vi "Biax24X setup.vi"() -> (0 "buffer size":i32=500000, 1 "Footer String":string, 2 "Channels, Hor load, Hor Disp, Vert Load, Vert Disp, LVDT1, LVDT2, LVDT3, LVDT4":string[](array[string])=["0", "1", "2", "3"], 3 "Number of Channels":i32, 4 "ASCII footer 2":bool, 5 "Device":i32=1, 6 "Channel Names":string[](array[string]), 8 "Header and Const.; Del, SR, #Scans, Write int":T1={"Delay"=-1.0, "Scan_Rate"=10000, "Number of scans"=10000, "Write time int (s)"=30} {"Delay" format="%.2f"})   [LabVIEW 2013]
doc: "This vi takes input from the operator: sets the scan rate, collects the length in inches, the sample diameter in inches, and the interchannel delay rate (default is -1.0) The vi puts out those constants along with the voltage limits for each of the data acquisition channels. The default settings are channel 0, 1 = confining and pore pressure transducer amplifiers, respectively, 0-5 volts; temperature transducer amplifier, 0-5 volts; dcdt +-3 volts (12.6 v/in); load cell after amplification: 12600 pounds force per volt."
uses:
  BiaxGlobals.vi
panel:
  in  "ASCII footer":bool=TRUE
  in  "String 23":string="Vert DCDT"
  in  "String 22":string="Vert LOAD"
  in  "String 21":string="Hor DCDT"
  in  "String 20":string="Hor LOAD"
  in  "String 19":string="Pc Disp"
  in  "String 18":string="Pc LOAD"
  in  "String 17":string="Ppa Disp"
  in  "String 16":string="Ppa LOAD"
  in  "Number of Channels":i32=4 min=1 max=8 step=1
  in  "Go on":bool
  in  "Delay":sgl=-1.0 format="%^.2e"
  out "Acquisition Rate \n(fixed at 10000 \nsamples/sec)":i32=10000
  out "Number of scans averaged for a single record output\n(while running Labview you can switch between 1, 10, 100, 1k, 10k samples/sec)":i32=10000
  in  "buffer size (500000 scans)":i32=500000
  out "write int":i32=30
  in  "Time interval to write to disk (seconds)\nNOTE: 30sec is optimal for 10 kHz sample rate":i32=30
  # "Press \"Go On\" when\nConstants are Entered\n\nDefault Delay setting \nis -1.0"
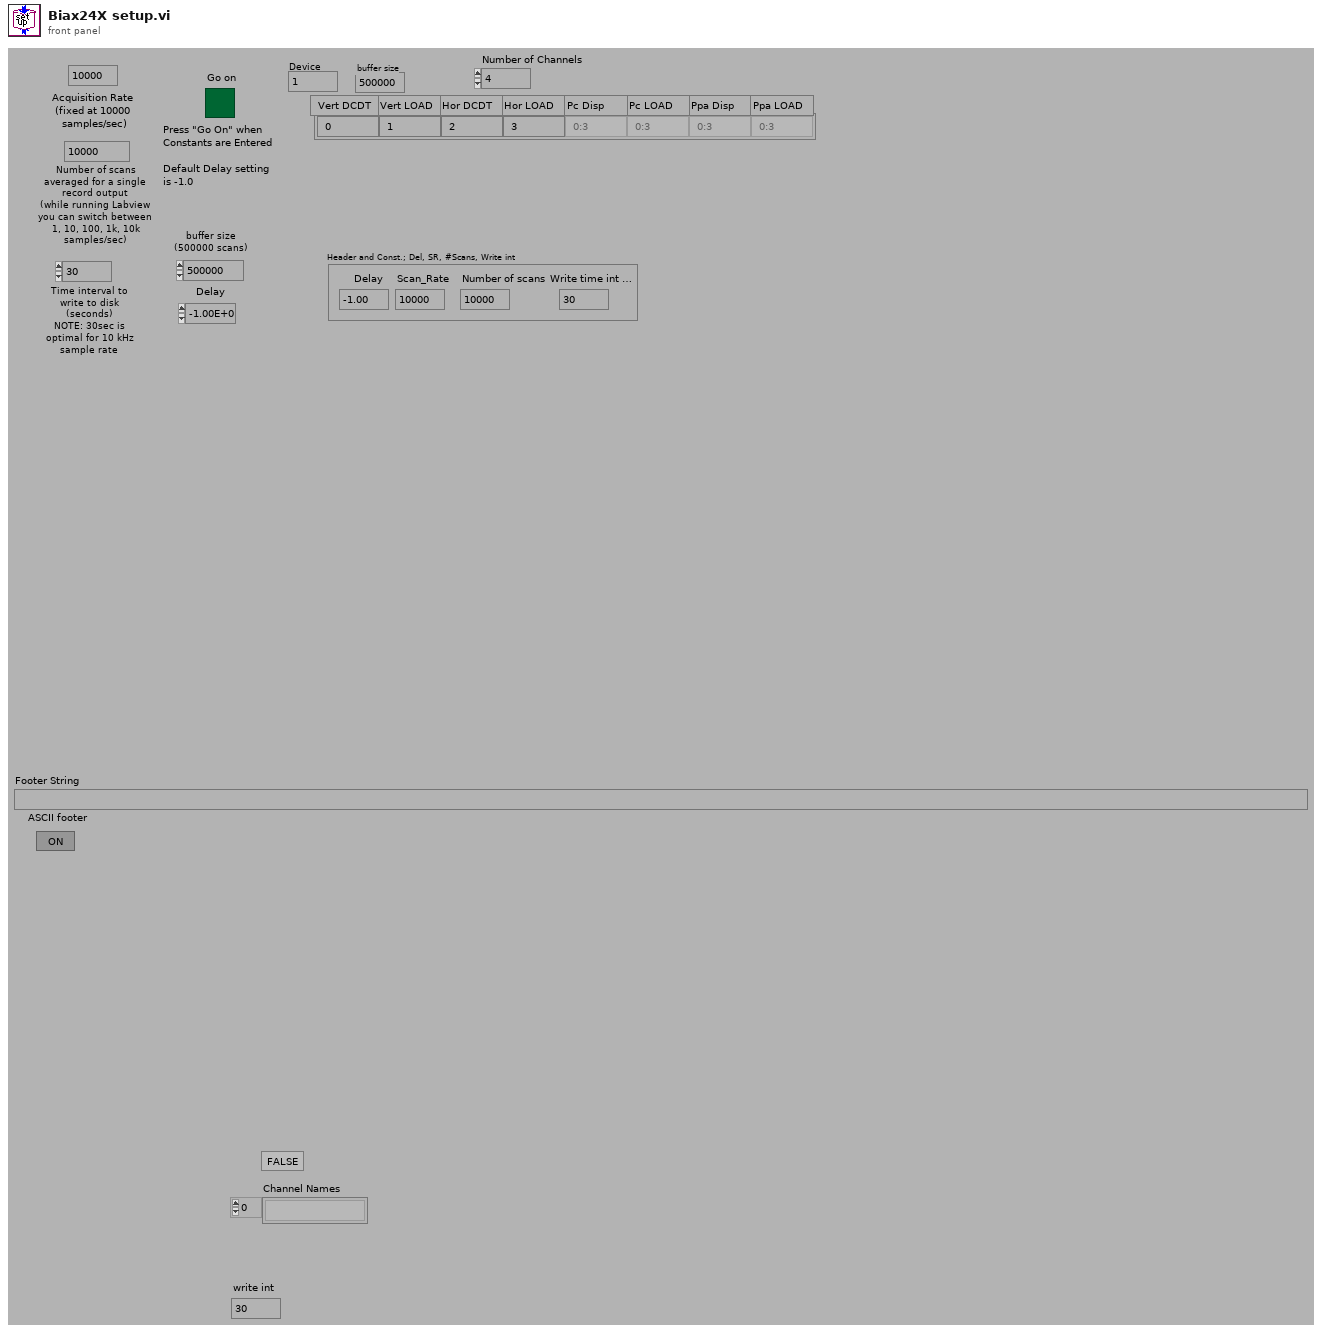
[diagram p1: front panel]
types:
  T1 = cluster{"Delay":dbl, "Scan_Rate":i32, "Number of scans":i32, "Write time int (s)":i32}
  T2 = cluster{"Delay":sgl, i32, i32, "Time interval to write to disk (seconds)\nNOTE: 30sec is optimal for 10 kHz sample rate":i32}
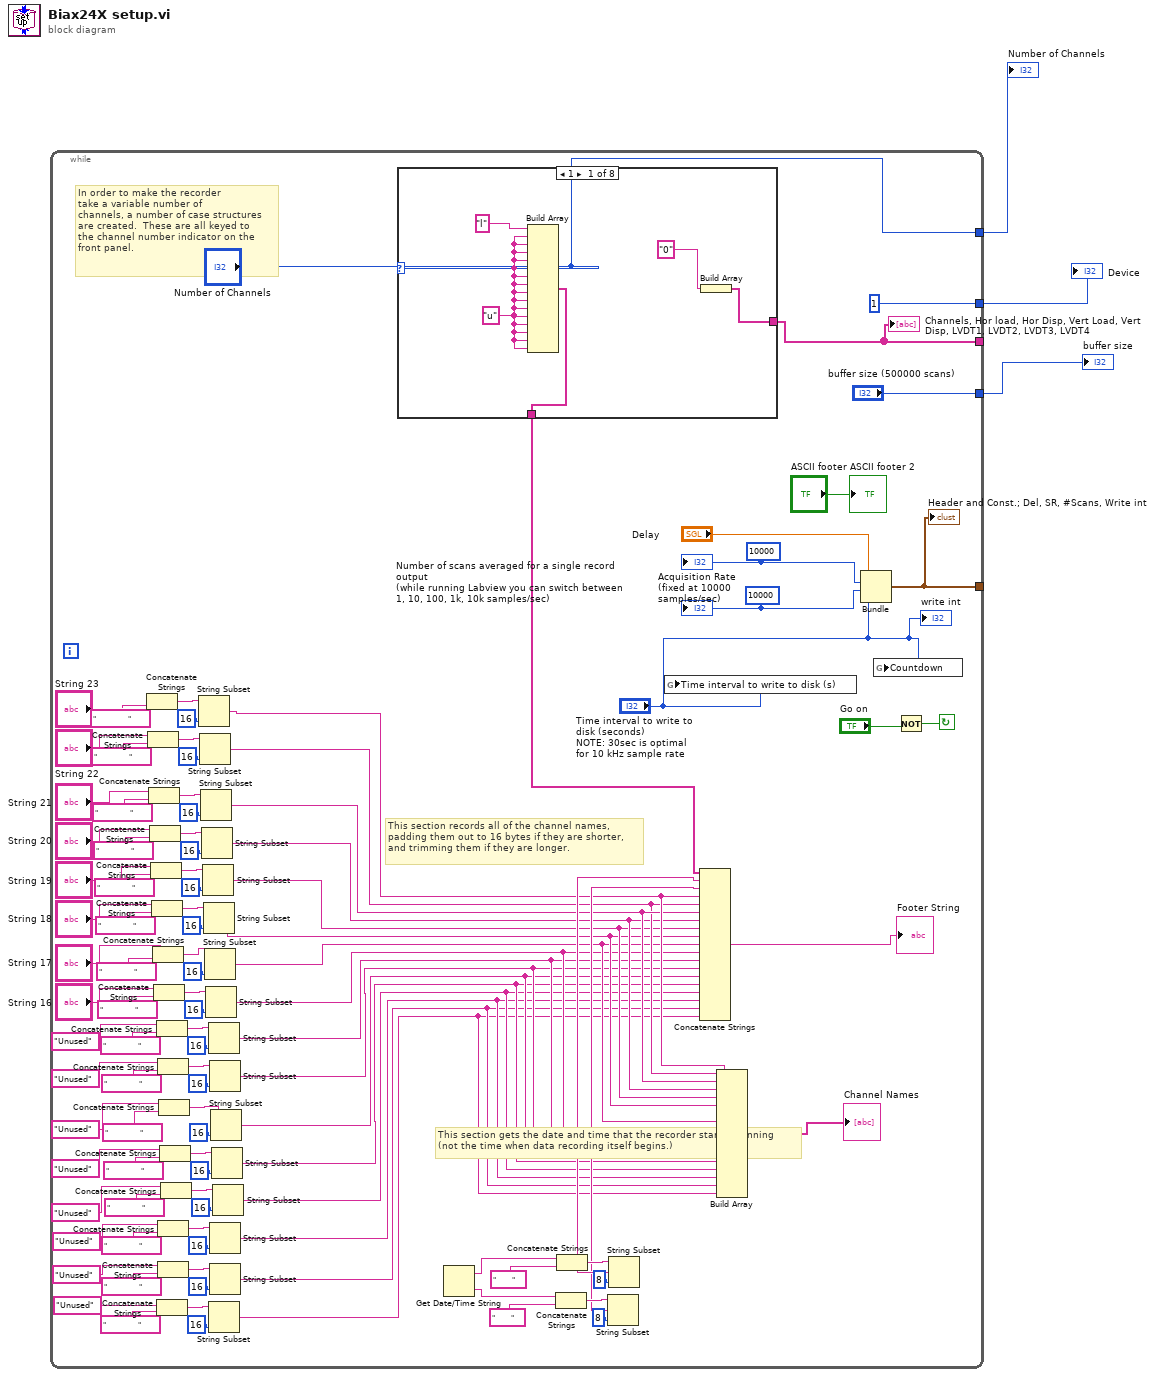
[diagram p0: block diagram]
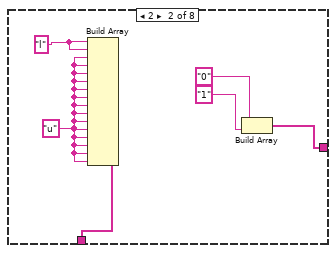
[diagram p2: hidden frame]
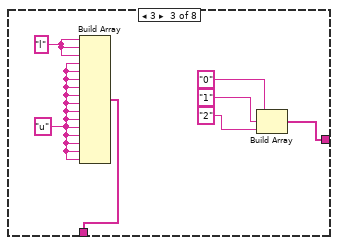
[diagram p3: hidden frame]
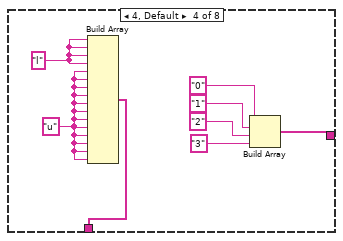
[diagram p4: hidden frame]
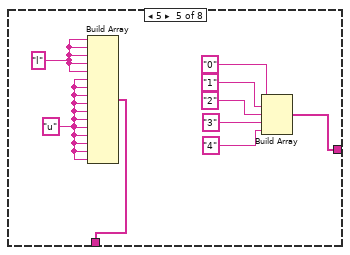
[diagram p5: hidden frame]
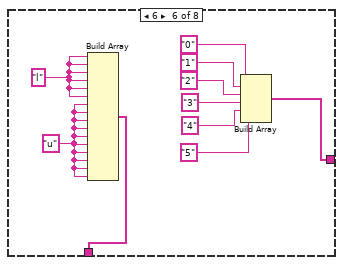
[diagram p6: hidden frame]
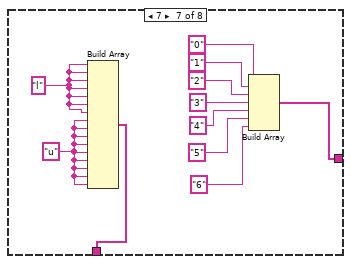
[diagram p7: hidden frame]
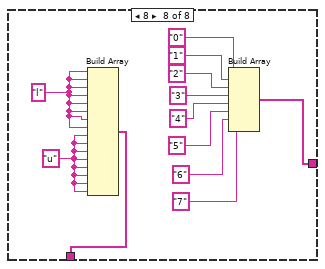
[diagram p8: hidden frame]
diagram:
  n1 = while {
    tunnel: ["buffer size (500000 scans)"] -> w3
    tunnel: [w99] -> _
    tunnel: [1] -> w2
    tunnel: [w98] -> _
    tunnel: ["Number of Channels"] -> w1
    stop <- w107 continue-if-true
    w101 = 10000
    w102 = 10000
    # "This section gets the date and time that the recorder started running \n(not the time when data recording itself begins.)"
    # "In order to make the recorder\ntake a variable number of\nchannels, a number of case structures\nare created.  These are all keyed to\nthe channel number indicator on the\nfront panel."
    # "This section records all of the channel names,\npadding them out to 16 bytes if they are shorter,\nand trimming them if they are longer."
    n2 = Concatenate Strings("String 23", "                ") -> (w95:string)
    n3 = Concatenate Strings("String 22", "                ") -> (w92:string)
    n4 = Concatenate Strings("String 21", "                ") -> (w89:string)
    n5 = Concatenate Strings("String 20", "                ") -> (w86:string)
    n6 = Concatenate Strings("String 19", "                ") -> (w83:string)
    n7 = Concatenate Strings("String 18", "                ") -> (w80:string)
    n8 = Concatenate Strings("String 17", "                ") -> (w77:string)
    n9 = Concatenate Strings("String 16", "                ") -> (w74:string)
    n10 = Concatenate Strings("Unused" ("String 24"), "                ") -> (w71:string)
    n11 = Concatenate Strings("Unused" ("String 24"), "                ") -> (w50:string)
    n12 = Concatenate Strings("Unused" ("String 24"), "                ") -> (w68:string)
    n13 = Concatenate Strings("Unused" ("String 24"), "                ") -> (w56:string)
    n14 = Concatenate Strings("Unused" ("String 24"), "                ") -> (w53:string)
    n15 = Concatenate Strings("Unused" ("String 24"), "                ") -> (w65:string)
    n16 = Concatenate Strings("Unused" ("String 24"), "                ") -> (w62:string)
    n17 = Concatenate Strings("Unused" ("String 24"), "                ") -> (w59:string)
    n18 = String Subset(string=w95, length (rest)=16 ("length (rest)")) -> (substring=w27:string)  [unwired: 1 in]
    n19 = String Subset(string=w92, length (rest)=16 ("length (rest)")) -> (substring=w25:string)  [unwired: 1 in]
    n20 = String Subset(string=w89, length (rest)=16 ("length (rest)")) -> (substring=w26:string)  [unwired: 1 in]
    n21 = String Subset(string=w86, length (rest)=16 ("length (rest)")) -> (substring=w24:string)  [unwired: 1 in]
    n22 = String Subset(string=w83, length (rest)=16 ("length (rest)")) -> (substring=w23:string)  [unwired: 1 in]
    n23 = String Subset(string=w80, length (rest)=16 ("length (rest)")) -> (substring=w22:string)  [unwired: 1 in]
    n24 = String Subset(string=w77, length (rest)=16 ("length (rest)")) -> (substring=w21:string)  [unwired: 1 in]
    n25 = String Subset(string=w74, length (rest)=16 ("length (rest)")) -> (substring=w20:string)  [unwired: 1 in]
    n26 = String Subset(string=w71, length (rest)=16 ("length (rest)")) -> (substring=w19:string)  [unwired: 1 in]
    n27 = String Subset(string=w50, length (rest)=16 ("length (rest)")) -> (substring=w12:string)  [unwired: 1 in]
    n28 = String Subset(string=w68, length (rest)=16 ("length (rest)")) -> (substring=w18:string)  [unwired: 1 in]
    n29 = String Subset(string=w56, length (rest)=16 ("length (rest)")) -> (substring=w14:string)  [unwired: 1 in]
    n30 = String Subset(string=w53, length (rest)=16 ("length (rest)")) -> (substring=w13:string)  [unwired: 1 in]
    n31 = String Subset(string=w65, length (rest)=16 ("length (rest)")) -> (substring=w17:string)  [unwired: 1 in]
    n32 = String Subset(string=w62, length (rest)=16 ("length (rest)")) -> (substring=w16:string)  [unwired: 1 in]
    n33 = String Subset(string=w59, length (rest)=16 ("length (rest)")) -> (substring=w15:string)  [unwired: 1 in]
    n34 = case shown="1" "Number of Channels" {
      tunnel: [w112 w117 w123 w134 w139 w147 w158 w168] -> w98
      tunnel: [w110 w114 w120 w127 w135 w145 w154 w167] -> w4
      frame 1 {
        w109 = "u" ("element")
        n35 = Build Array("l", w109, w109, w109, w109, w109, w109, w109, w109, w109, w109, w109, w109, w109, w109, w109) -> (w110:string[])
        n36 = Build Array("0") -> (w112:string[])
      }
      frame 2 {
        w115 = "u" ("element")
        w116 = "l"
        n37 = Build Array(w116, w116, w115, w115, w115, w115, w115, w115, w115, w115, w115, w115, w115, w115, w115, w115) -> (w114:string[])
        n38 = Build Array("0", "1") -> (w117:string[])
      }
      frame 3 {
        w121 = "u" ("element")
        w122 = "l"
        n39 = Build Array(w122, w122, w122, w121, w121, w121, w121, w121, w121, w121, w121, w121, w121, w121, w121, w121) -> (w120:string[])
        n40 = Build Array("0", "1", "2") -> (w123:string[])
      }
      frame 4, Default {
        w128 = "u" ("element")
        w129 = "l"
        n41 = Build Array(w129, w129, w129, w129, w128, w128, w128, w128, w128, w128, w128, w128, w128, w128, w128, w128) -> (w127:string[])
        n42 = Build Array("0", "1", "2", "3") -> (w134:string[])
      }
      frame 5 {
        w136 = "u" ("element")
        w137 = "l"
        n43 = Build Array(w137, w137, w137, w137, w137, w136, w136, w136, w136, w136, w136, w136, w136, w136, w136, w136) -> (w135:string[])
        n44 = Build Array("0", "1", "2", "3", "4") -> (w139:string[])
      }
      frame 6 {
        w144 = "u" ("element")
        w146 = "l"
        n45 = Build Array(w146, w146, w146, w146, w146, w146, w144, w144, w144, w144, w144, w144, w144, w144, w144, w144) -> (w145:string[])
        n46 = Build Array("0", "1", "2", "3", "4", "5") -> (w147:string[])
      }
      frame 7 {
        w155 = "u" ("element")
        w156 = "l"
        n47 = Build Array(w156, w156, w156, w156, w156, w156, w156, w155, w155, w155, w155, w155, w155, w155, w155, w155) -> (w154:string[])
        n48 = Build Array("0", "1", "2", "3", "4", "5", "6") -> (w158:string[])
      }
      frame 8 {
        w165 = "u" ("element")
        w166 = "l"
        n49 = Build Array(w166, w166, w166, w166, w166, w166, w166, w166, w165, w165, w165, w165, w165, w165, w165, w165) -> (w167:string[])
        n50 = Build Array("0", "1", "2", "3", "4", "5", "6", "7") -> (w168:string[])
      }
    }
    "Channels, Hor load, Hor Disp, Vert Load, Vert Disp, LVDT1, LVDT2, LVDT3, LVDT4" <- w98
    n51 = Get Date/Time String() -> (date string=w31:string, time string=w30:string)  [unwired: 3 in]
    n52 = Concatenate Strings(w30, "        ") -> (w33:string)
    n53 = Concatenate Strings(w31, "        ") -> (w36:string)
    n54 = String Subset(string=w33, length (rest)=8 ("length (rest)")) -> (substring=w28:string)  [unwired: 1 in]
    n55 = String Subset(string=w36, length (rest)=8 ("length (rest)")) -> (substring=w29:string)  [unwired: 1 in]
    n56 = global write "BiaxGlobals.vi" "Time interval to write to disk (s)"("Time interval to write to disk (seconds)\nNOTE: 30sec is optimal for 10 kHz sample rate") -> ()
    n57 = Concatenate Strings(w4, w29, w28, w27, w25, w26, w24, w23, w22, w21, w20, w19, w18, w17, w16, w15, w14, w13, w12) -> (→"Footer String":string)
    n58 = Build Array(w27, w25, w26, w24, w23, w22, w21, w20, w19, w18, w17, w16, w15, w14, w13, w12) -> (→"Channel Names":string[])
    n59 = Bundle("Delay"="Delay", w102, w101, "Time interval to write to disk (seconds)\nNOTE: 30sec is optimal for 10 kHz sample rate"="Time interval to write to disk (seconds)\nNOTE: 30sec is optimal for 10 kHz sample rate") -> (w99:T2)  [unwired: 1 in]
    "Header and Const.; Del, SR, #Scans, Write int" <- w99
    n60 = global write "BiaxGlobals.vi" "Countdown"("Time interval to write to disk (seconds)\nNOTE: 30sec is optimal for 10 kHz sample rate") -> ()
    n61 = Not(x="Go on") -> (.not. x?=w107:bool)
    "Acquisition Rate \n(fixed at 10000 \nsamples/sec)" <- w102
    "Number of scans averaged for a single record output\n(while running Labview you can switch between 1, 10, 100, 1k, 10k samples/sec)" <- w101
    "write int" <- "Time interval to write to disk (seconds)\nNOTE: 30sec is optimal for 10 kHz sample rate"
    "ASCII footer 2" <- "ASCII footer"
  }
  "Device" <- w2
  "buffer size" <- w3
  "Number of Channels" <- w1
